vi "Create Key Treshold Map.vi"(8 "error in (no error)":errorcluster, 10 "Tresholds":refnum<class "1D Array s32.lvclass">, 11 "Key Map Primitive":refnum<class "2D Array u32.lvclass">) -> (0 "error out":errorcluster, 3 "Key Treshold Map":refnum<class "1D Array u32.lvclass">)   [LabVIEW 2024, in "G2CPU Line Profile.lvlib"]
uses:
  G2CPU Line Profile.lvlib
  <vilib>/Natan Biesmans/G2CPU GPU and CPU HPC Toolkit/G2CPU Libraries/Arrays/1DArray/u32/1D Array u32.lvclass
  C:/Program Files/National Instruments/LabVIEW 2025/vi.lib/Natan Biesmans/G2CPU GPU and CPU HPC Toolkit/G2CPU Libraries/Arrays/Array/Array Prototype.lvclass
  <vilib>/Natan Biesmans/G2CPU GPU and CPU HPC Toolkit/G2CPU Libraries/Arrays/2DArray/u32/2D Array u32.lvclass
  <vilib>/Natan Biesmans/G2CPU GPU and CPU HPC Toolkit/G2CPU Libraries/Arrays/1DArray/s32/1D Array s32.lvclass
  dfc296d6-09e9-49d4-b6a7-8f7cba126448.vi
  0e00f3ea-295d-46eb-a73e-b789dd041baa.vi
  df6f60ea-b988-4197-85ce-3a8efc5252c5.vi
  a54cd3ce-7813-4a8a-b799-036ee925c274.vi
  dfc296d6-09e9-49d4-b6a7-8f7cba126448.vi/d8e2d9cc-c923-495e-b121-b6b84788c73f.vi
  dfc296d6-09e9-49d4-b6a7-8f7cba126448.vi/345e91f0-9a5e-4de4-af9c-133346717e4a.vi
  0e00f3ea-295d-46eb-a73e-b789dd041baa.vi/5793b77b-c002-4ebf-9075-685617c95341.vi
  0e00f3ea-295d-46eb-a73e-b789dd041baa.vi/2ed3ef86-c00d-4d71-b84c-20267a6dfcf9.vi
  df6f60ea-b988-4197-85ce-3a8efc5252c5.vi/e9bebd79-1c27-4fc1-b91f-30516104c7f0.vi
  a54cd3ce-7813-4a8a-b799-036ee925c274.vi/7467a0f1-0650-4e63-b635-b3d2b2ec9a4e.vi
  a54cd3ce-7813-4a8a-b799-036ee925c274.vi/8ee11bc3-5ef5-497e-97f0-8db2b3aaa149.vi
  a54cd3ce-7813-4a8a-b799-036ee925c274.vi/c7af9698-5e3c-4e11-95da-3024075b67d2.vi
  0e00f3ea-295d-46eb-a73e-b789dd041baa.vi/5793b77b-c002-4ebf-9075-685617c95341.vi/3e802c67-fb96-46a3-ae13-4994a8508b4f.vi
  0e00f3ea-295d-46eb-a73e-b789dd041baa.vi/5793b77b-c002-4ebf-9075-685617c95341.vi/5a50fc67-79e7-4972-80c2-92243cd53dd4.vi
  0e00f3ea-295d-46eb-a73e-b789dd041baa.vi/2ed3ef86-c00d-4d71-b84c-20267a6dfcf9.vi/730f6c57-5c0b-4ee9-b61e-75067b25222b.vi
  0e00f3ea-295d-46eb-a73e-b789dd041baa.vi/2ed3ef86-c00d-4d71-b84c-20267a6dfcf9.vi/096b8799-7810-404e-baca-ba9279cec4bd.vi
  0e00f3ea-295d-46eb-a73e-b789dd041baa.vi/2ed3ef86-c00d-4d71-b84c-20267a6dfcf9.vi/0f1a5a47-bcc5-4796-ac31-8dfcfbc0d7d1.vi
  0e00f3ea-295d-46eb-a73e-b789dd041baa.vi/2ed3ef86-c00d-4d71-b84c-20267a6dfcf9.vi/89f12e17-3330-4b72-ad8f-8dd636660732.vi
  <vilib>/Natan Biesmans/G2CPU GPU and CPU HPC Toolkit/G2CPU Libraries/Arrays/Array/G2CPU Get Array Pointer.vi
  <vilib>/Natan Biesmans/G2CPU GPU and CPU HPC Toolkit/ArrayFire Driver/VIs/cast.vi
  <vilib>/Natan Biesmans/G2CPU GPU and CPU HPC Toolkit/G2CPU Libraries/Arrays/Array/G2CPU Set Array Pointer.vi
  <vilib>/Natan Biesmans/G2CPU GPU and CPU HPC Toolkit/G2CPU Libraries/Arrays/Array/G2CPU Unlock Array.vi
  <vilib>/Natan Biesmans/G2CPU GPU and CPU HPC Toolkit/G2CPU Libraries/Arrays/Array/G2CPU Release Array.vi
  <vilib>/Natan Biesmans/G2CPU GPU and CPU HPC Toolkit/G2CPU Libraries/Arrays/SubVI/Lock Arrays.vi
  <vilib>/Natan Biesmans/G2CPU GPU and CPU HPC Toolkit/G2CPU Libraries/Arrays/SubVI/is 2D.vi
  <vilib>/Natan Biesmans/G2CPU GPU and CPU HPC Toolkit/ArrayFire Driver/VIs/add.vi
  <vilib>/Natan Biesmans/G2CPU GPU and CPU HPC Toolkit/G2CPU Libraries/Arrays/Array/G2CPU Lock Array.vi
  <vilib>/Natan Biesmans/G2CPU GPU and CPU HPC Toolkit/ArrayFire Driver/VIs/transpose.vi
  <vilib>/Natan Biesmans/G2CPU GPU and CPU HPC Toolkit/ArrayFire Driver/VIs/flat.vi
  <vilib>/Natan Biesmans/G2CPU GPU and CPU HPC Toolkit/G2CPU Libraries/Arrays/Array/Array Prototype.lvclass
  <vilib>/Natan Biesmans/G2CPU GPU and CPU HPC Toolkit/G2CPU Libraries/Arrays/DataTypes/U32/U32.lvclass
  <vilib>/Natan Biesmans/G2CPU GPU and CPU HPC Toolkit/G2CPU Libraries/Arrays/2DArray/2D Array Prototype.lvclass
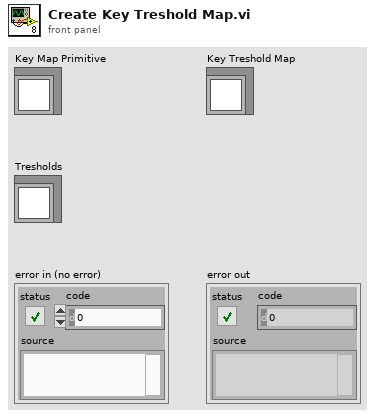
[diagram p1: front panel]
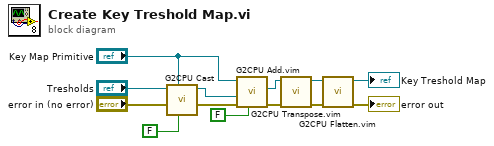
[diagram p0: block diagram]
diagram:
  n1 = call "G2CPU Cast"("Auto Release Low (Enabled)"=FALSE, "Datatype Prototype"="Key Map Primitive", "error in (no error)"="error in (no error)", "Array In"="Tresholds") -> ("error out"=w5:errorcluster, "Array Out"=w2:refnum<class "2D Array u32.lvclass">)  [unwired: 6 in]
  n2 = call "G2CPU Add.vim"("Auto Release lhs (Enabled)"=FALSE, "error in (no error)"=w5, "Array rhs"=w2, "Array lhs"="Key Map Primitive") -> ("error out"=w7:errorcluster, "Array Result"=w6:refnum<class "2D Array u32.lvclass">)  [unwired: 6 in]
  n3 = call "G2CPU Transpose.vim"("error in (no error)"=w7, "Array In"=w6) -> ("error out"=w9:errorcluster, "Array out"=w8:refnum<class "2D Array u32.lvclass">)  [unwired: 8 in]
  n4 = call "G2CPU Flatten.vim"("error in (no error)"=w9, "Array In"=w8) -> ("error out"=→"error out":errorcluster, "Array out"=→"Key Treshold Map":refnum<class "1D Array u32.lvclass">)  [unwired: 8 in]
